vi "publishAck.vi"(8 "error in (no error)":errorcluster, 10 "AckType":T1, 11 "MonoCommunicator in":refnum<class "MonoCommunicator.lvclass">) -> (0 "error out":errorcluster, 3 "MonoCommunicator out":refnum<class "MonoCommunicator.lvclass">)   [LabVIEW 2016, in "MonoCommunicator.lvclass"]
uses:
  MonoCommunicator.lvclass
  Typedefs/AckType.ctl
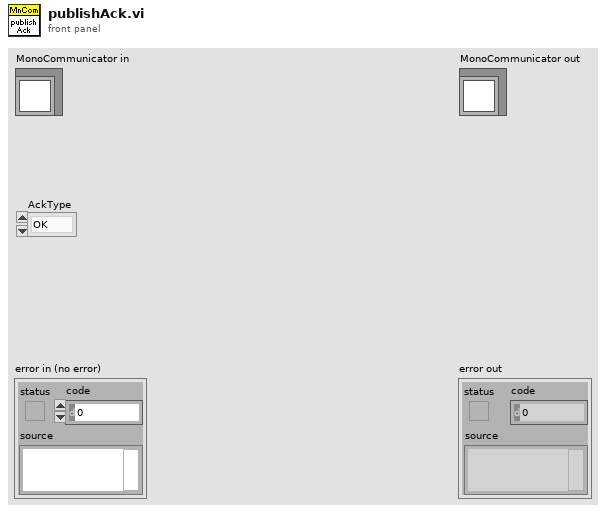
[diagram p1: front panel]
types:
  T1 = typedef "AckType.ctl" = enum16{"OK", "OutOfRange", "Unknown", "Busy", "Rejected"}
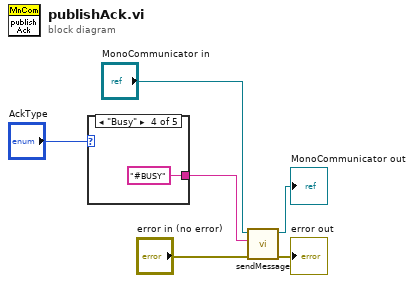
[diagram p0: block diagram]
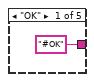
[diagram p2: hidden frame]
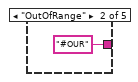
[diagram p3: hidden frame]
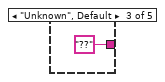
[diagram p4: hidden frame]
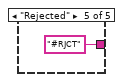
[diagram p5: hidden frame]
diagram:
  n1 = case shown="\"Busy\"" "AckType" {
    tunnel: ["#OK" "#OUR" "??" "#BUSY" "#RJCT"] -> w1
    frame "OK" {
    }
    frame "OutOfRange" {
    }
    frame "Unknown", Default {
    }
    frame "Busy" {
    }
    frame "Rejected" {
    }
  }
  n2 = call "sendMessage.vi"("error in (no error)"="error in (no error)", "message"=w1, "MonoCommunicator in"="MonoCommunicator in") -> ("error out"=→"error out":errorcluster, "MonoCommunicator out"=→"MonoCommunicator out":refnum<class "MonoCommunicator.lvclass">)  [unwired: 7 in]
